vi "Motor planner.vi"(7 "Number of cycles":i32, 8 "Error In":errorcluster, 10 "Command planner":T2(array[cluster]), 11 "VISA in":refnum<visa-resource-name>) -> (0 "Error Out":errorcluster, 3 "VISA out":refnum<visa-resource-name>)   [LabVIEW 2014]
uses:
  Typedef/Process scheduler - Commands.ctl
  Typedef/Move type.ctl
  Motor manager.lvlib
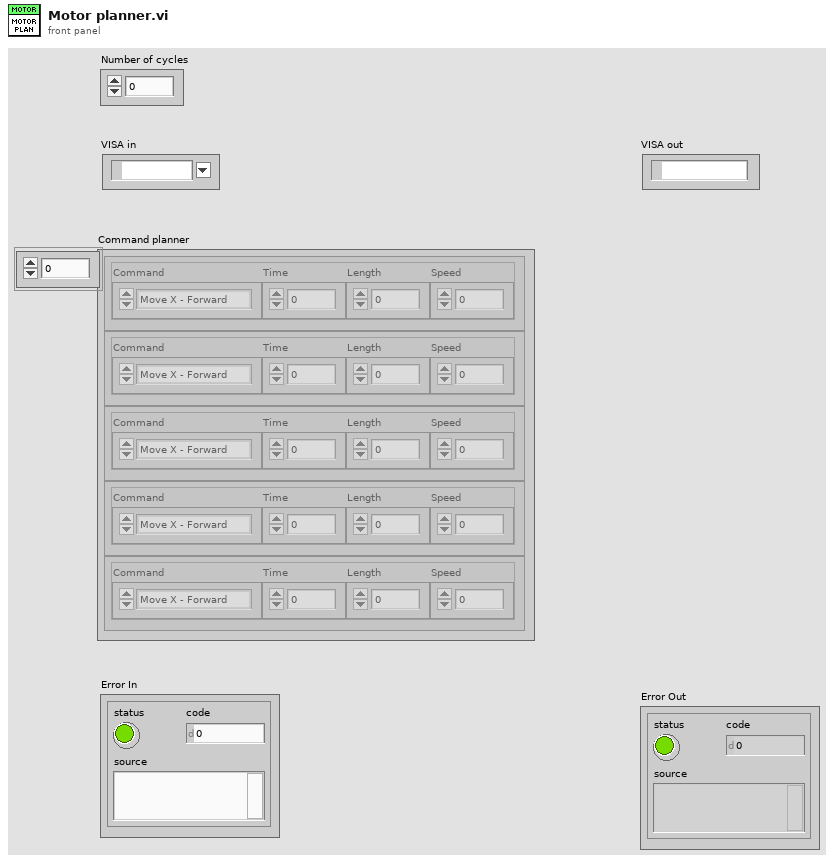
[diagram p1: front panel]
types:
  T1 = typedef "Process scheduler - Commands.ctl" = enum16{"None", "Move X - Forward", "Move X - Backward", "Move Y - Forward", "Move Y - Backward", "Wait X", "Wait Y", "Change speed X", "Change speed Y"}
  T2 = cluster{"Command":T1, "Time":sgl, "Length":sgl, "Speed":u32}[]
  T3 = typedef "Motor manager.lvlib/Move type.ctl" = enum16{"Move forward", "Move backward", "Cycle (forward first)", "Cycle (backward first)"}
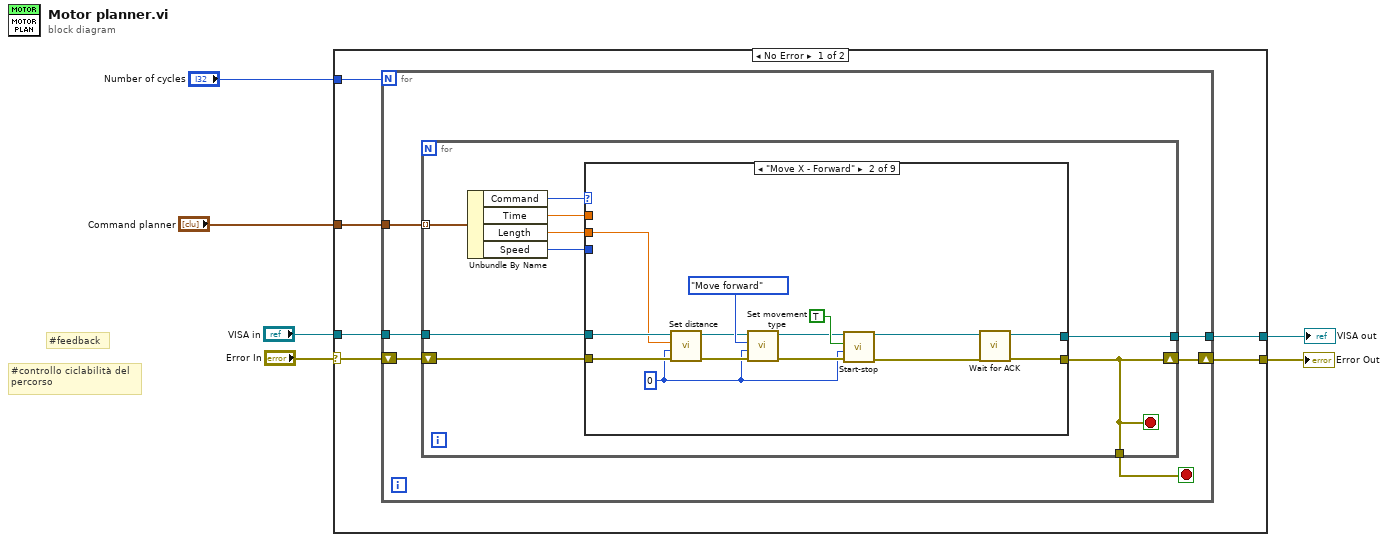
[diagram p0: block diagram]
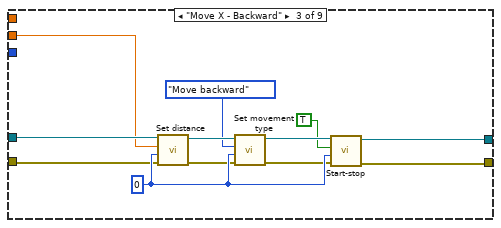
[diagram p3: hidden frame]
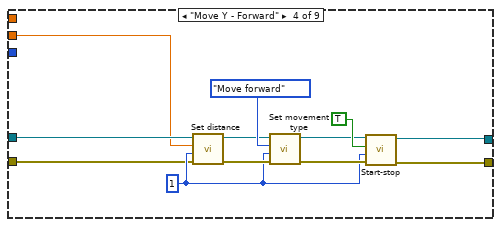
[diagram p4: hidden frame]
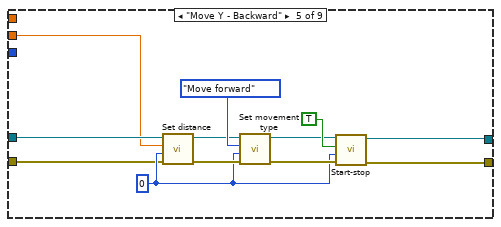
[diagram p5: hidden frame]
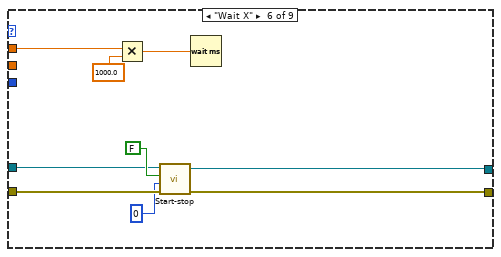
[diagram p6: hidden frame]
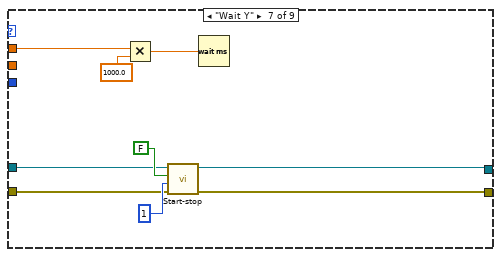
[diagram p7: hidden frame]
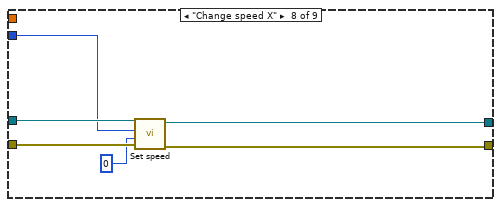
[diagram p8: hidden frame]
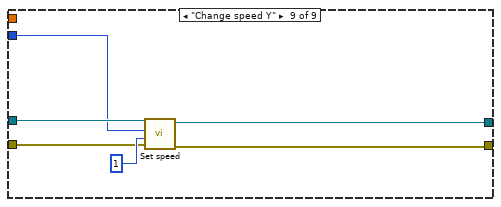
[diagram p9: hidden frame]
diagram:
  # "#controllo ciclabilità del\npercorso"
  # "#feedback"
  n1 = case shown="No Error" "Error In" {
    selector: "Error In" -> [w12 w111]
    tunnel: [w11 w111] -> w4
    tunnel: "Number of cycles" -> [w10 _]
    tunnel: "Command planner" -> [w9 _]
    tunnel: "VISA in" -> [w8 w110]
    tunnel: [w7 w110] -> w1
    frame No Error {
      n2 = for {
        N: w10 -> [_]
        tunnel: w9 -> [w16]
        tunnel: w8 -> [w14]
        tunnel: [w13] -> w7
        shift-right: [w17] -> w11
        shift-left: w12 -> [w18]
        stop <- w15 stop-if-true
        n3 = for {
          tunnel: w16 -> [w27] mode=indexing
          tunnel: [w24] -> w15
          tunnel: w14 -> [w20]
          tunnel: [w19] -> w13
          shift-right: [w24] -> w17
          shift-left: w18 -> [w25]
          stop <- w24 stop-if-true
          n4 = Unbundle By Name(w27) -> ("Command"=w26:T1, "Time"=w23:sgl, "Length"=w22:sgl, "Speed"=w21:u32)
          n5 = case shown="\"Move X - Forward\"" w26 {
            tunnel: w25 -> [w29 w43 w48 w60 w72 w86 w91 w102 w107]
            tunnel: [w29 w32 w45 w56 w68 w80 w89 w98 w104] -> w24
            tunnel: w23 -> [_ _ _ _ _ w84 w93 _ _]
            tunnel: w22 -> [_ w35 w46 w58 w70 _ _ _ _]
            tunnel: w21 -> [_ _ _ _ _ _ _ w101 w106]
            tunnel: w20 -> [w28 w42 w47 w59 w71 w87 w92 w103 w108]
            tunnel: [w28 w31 w44 w57 w69 w81 w90 w99 w105] -> w19
            frame "None", Default {
            }
            frame "Move X - Forward" {
              w34 = u8 0 ("Motor index")
              n6 = call "Set distance.vi"("Error In"=w43, "Motor index"=w34, "Travel distance"=w35, "VISA resource in"=w42) -> ("Error Out"=w40:errorcluster, "VISA resource out"=w39:refnum<visa-resource-name>)  [unwired: 6 in]
              n7 = call "Set movement type.vi"("Error In"=w40, "Motor index"=w34, "Movement type"=Move_type."Move forward", "VISA resource in"=w39) -> ("Error Out"=w36:errorcluster, "VISA resource out"=w37:refnum<visa-resource-name>)  [unwired: 6 in]
              n8 = call "Start-stop.vi"("Error In"=w36, "Motor index"=w34, "Go"=TRUE, "VISA resource in"=w37) -> ("Error Out"=w33:errorcluster, "VISA resource out"=w30:refnum<visa-resource-name>)  [unwired: 6 in]
              n9 = call "Wait for ACK.vi"("Error In"=w33, "VISA in"=w30) -> ("Error Out"=w32:errorcluster, "VISA out"=w31:refnum<visa-resource-name>)  [unwired: 7 in, 1 out]
            }
            frame "Move X - Backward" {
              w55 = u8 0 ("Motor index")
              n10 = call "Set distance.vi"("Error In"=w48, "Motor index"=w55, "Travel distance"=w46, "VISA resource in"=w47) -> ("Error Out"=w50:errorcluster, "VISA resource out"=w51:refnum<visa-resource-name>)  [unwired: 6 in]
              n11 = call "Set movement type.vi"("Error In"=w50, "Motor index"=w55, "Movement type"=Move_type."Move backward", "VISA resource in"=w51) -> ("Error Out"=w54:errorcluster, "VISA resource out"=w53:refnum<visa-resource-name>)  [unwired: 6 in]
              n12 = call "Start-stop.vi"("Error In"=w54, "Motor index"=w55, "Go"=TRUE, "VISA resource in"=w53) -> ("Error Out"=w45:errorcluster, "VISA resource out"=w44:refnum<visa-resource-name>)  [unwired: 6 in]
            }
            frame "Move Y - Forward" {
              w61 = u8 1 ("Motor index")
              n13 = call "Set distance.vi"("Error In"=w60, "Motor index"=w61, "Travel distance"=w58, "VISA resource in"=w59) -> ("Error Out"=w66:errorcluster, "VISA resource out"=w65:refnum<visa-resource-name>)  [unwired: 6 in]
              n14 = call "Set movement type.vi"("Error In"=w66, "Motor index"=w61, "Movement type"=Move_type."Move forward", "VISA resource in"=w65) -> ("Error Out"=w62:errorcluster, "VISA resource out"=w63:refnum<visa-resource-name>)  [unwired: 6 in]
              n15 = call "Start-stop.vi"("Error In"=w62, "Motor index"=w61, "Go"=TRUE, "VISA resource in"=w63) -> ("Error Out"=w56:errorcluster, "VISA resource out"=w57:refnum<visa-resource-name>)  [unwired: 6 in]
            }
            frame "Move Y - Backward" {
              w73 = u8 0 ("Motor index")
              n16 = call "Set distance.vi"("Error In"=w72, "Motor index"=w73, "Travel distance"=w70, "VISA resource in"=w71) -> ("Error Out"=w78:errorcluster, "VISA resource out"=w77:refnum<visa-resource-name>)  [unwired: 6 in]
              n17 = call "Set movement type.vi"("Error In"=w78, "Motor index"=w73, "Movement type"=Move_type."Move forward", "VISA resource in"=w77) -> ("Error Out"=w74:errorcluster, "VISA resource out"=w75:refnum<visa-resource-name>)  [unwired: 6 in]
              n18 = call "Start-stop.vi"("Error In"=w74, "Motor index"=w73, "Go"=TRUE, "VISA resource in"=w75) -> ("Error Out"=w68:errorcluster, "VISA resource out"=w69:refnum<visa-resource-name>)  [unwired: 6 in]
            }
            frame "Wait X" {
              n19 = Multiply(x=w84, y=sgl 1000.0) -> (x*y=w82:sgl)
              n20 = call "Start-stop.vi"("Error In"=w86, "Motor index"=u8 0, "Go"=FALSE, "VISA resource in"=w87) -> ("Error Out"=w80:errorcluster, "VISA resource out"=w81:refnum<visa-resource-name>)  [unwired: 6 in]
              n21 = Wait (ms)(milliseconds to wait=w82) -> ()  [unwired: 1 out]
            }
            frame "Wait Y" {
              n22 = Multiply(x=w93, y=sgl 1000.0) -> (x*y=w94:sgl)
              n23 = call "Start-stop.vi"("Error In"=w91, "Motor index"=u8 1, "Go"=FALSE, "VISA resource in"=w92) -> ("Error Out"=w89:errorcluster, "VISA resource out"=w90:refnum<visa-resource-name>)  [unwired: 6 in]
              n24 = Wait (ms)(milliseconds to wait=w94) -> ()  [unwired: 1 out]
            }
            frame "Change speed X" {
              n25 = call "Set speed.vi"("Error In"=w102, "Motor index"=u8 0, "Speed"=w101, "VISA resource in"=w103) -> ("Error Out"=w98:errorcluster, "VISA resource out"=w99:refnum<visa-resource-name>)  [unwired: 6 in]
            }
            frame "Change speed Y" {
              n26 = call "Set speed.vi"("Error In"=w107, "Motor index"=u8 1, "Speed"=w106, "VISA resource in"=w108) -> ("Error Out"=w104:errorcluster, "VISA resource out"=w105:refnum<visa-resource-name>)  [unwired: 6 in]
            }
          }
        }
      }
    }
    frame Error {
    }
  }
  "Error Out" <- w4
  "VISA out" <- w1
